vi "NT Read Generic Value.vi"(8 "error in":errorcluster, 11 "Name":string="Boolean") -> (0 "error out":errorcluster, 3 "Field Value":T1)   [LabVIEW 2017]
doc: "Return the tagged cluster data for then named entry."
uses:
  <vilib>/Rock Robotics/Network Tables/Field Data.ctl
  <vilib>/Rock Robotics/Network Tables/Field Type.ctl
  <vilib>/Rock Robotics/Network Tables/Sequence.ctl
  <vilib>/Rock Robotics/Network Tables/Make Table Operation.ctl
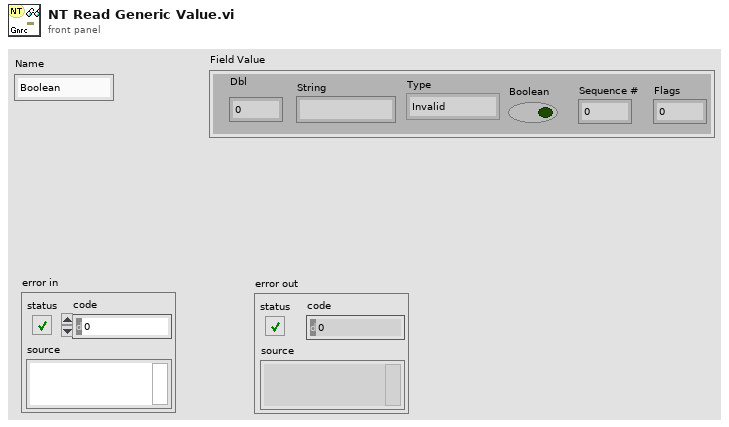
[diagram p1: front panel]
types:
  T1 = typedef "Field Data.ctl" = cluster{"Dbl":dbl, "String":string, "Type":T2, "Boolean":bool, "Sequence #":T3, "Flags":u8}
  T2 = typedef "Field Type.ctl" = enum8{"Invalid", "Bool", "Numeric", "String", "Raw", "Boolean Array", "Numeric Array", "String Array", "RPC"}
  T3 = typedef "Sequence.ctl" = u16
  T4 = typedef "Make Table Operation.ctl" = enum16{"Get or Add Field", "Get Field or Add Temp", "Replace Temp ID", "Get Field ID - No Add", "Get Table Field IDs", "Get Field ID Info", "Move Field to Temp", "Validate", "Remove Field", "Remove All"}
  T5 = typedef "Field ID.ctl" = i32
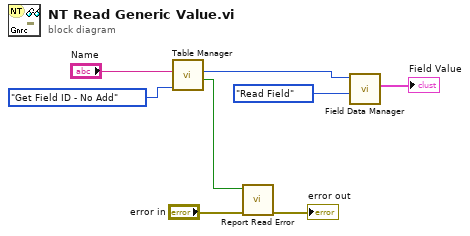
[diagram p0: block diagram]
diagram:
  n1 = call <vilib>:"Table Manager.vi"("Operation"=Make_Table_Operation."Get Field ID - No Add", "Entry Name"="Name") -> ("Success"=w1:bool, "Entry ID"=w6:T5)  [unwired: 6 in, 2 out]
  n2 = call <vilib>:"Report Read Error.vi"("error in (no error)"="error in", "Success"=w1) -> ("error out"=→"error out":errorcluster)  [unwired: 9 in]
  n3 = call <vilib>:"Field Data Manager.vi"("Operation"=enum16{"Update Field", "Read Field"}."Read Field", "Field ID"=w6) -> ("Field Value Out"=→"Field Value":T1)  [unwired: 8 in, 1 out]
